vi "GetScanPos.vi"(8 "error in (no error)":errorcluster caption="entrée d'erreur (pas d'erreur)", 10 "ParIndex":i32, 11 "Experiment en entrée":refnum<class "Experiment.lvclass"> caption="DNL_LabVIEW Object in") -> (0 "error out":errorcluster caption="sortie d'erreur", 2 "ScanTable":dbl[](array[numeric]), 3 "Experiment en sortie":refnum<class "Experiment.lvclass"> caption="DNL_LabVIEW Object out")   [LabVIEW 2019, in "Experiment.lvclass"]
uses:
  Experiment.lvclass
  Experiment.lvclass/Experiment.ctl
  DevicesClass/BaseDevice/BaseDevice.lvclass
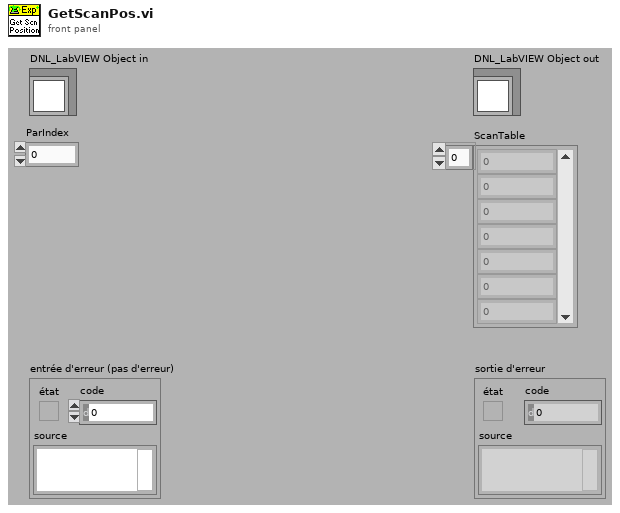
[diagram p1: front panel]
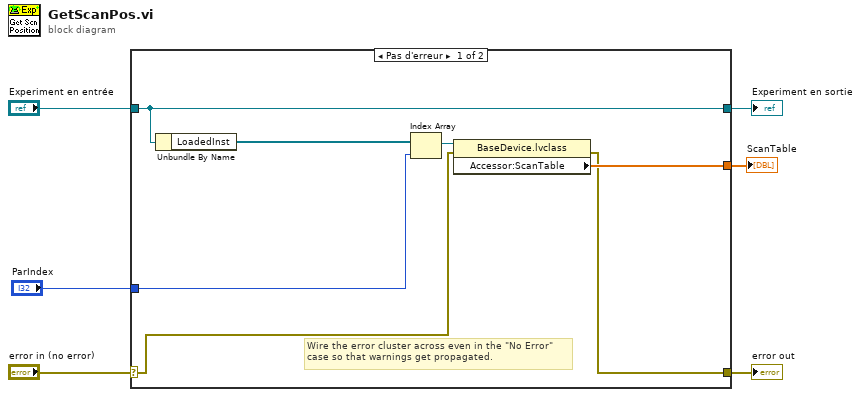
[diagram p0: block diagram]
diagram:
  n1 = case shown="Pas d'erreur" "error in (no error)" {
    selector: "error in (no error)" -> [w8 w15]
    tunnel: [w7 w15] -> w5
    tunnel: [w13 w14] -> w3
    tunnel: "Experiment en entrée" -> [w13 w14]
    tunnel: "ParIndex" -> [w9 _]
    tunnel: [w10 _] -> w1
    frame No Error {
      # "Wire the error cluster across even in the \"No Error\"\ncase so that warnings get propagated."
      n2 = Unbundle By Name(w13) -> ("LoadedInst"=w12:refnum<class "BaseDevice.lvclass">[])
      n3 = Index Array(array=w12, index=w9) -> (element=w11:refnum<class "BaseDevice.lvclass">)
      n4 = property class="BaseDevice.lvclass"(reference=w11, error in=w8) -> (error out=w7:errorcluster, "Accessor:ScanTable"=w10:dbl[])  [unwired: 1 out]
    }
    frame Error {
    }
  }
  "error out" <- w5
  "Experiment en sortie" <- w3
  "ScanTable" <- w1
